vi "SetGain.vi"(10 "Gain":refnum<vi>, 11 ".NET Refnum in":refnum<k24>) -> (3 ".NET Refnum out":refnum<k24>)   [LabVIEW 2018]
uses:
  D:/SVN/PM/sdk/AppSamples/LabVIEWSamples/trunk/Release/2018/Dependencies/PVCamNET.dll
  Dependencies/PVCamNET.dll
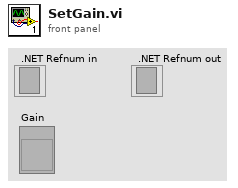
[diagram p1: front panel]
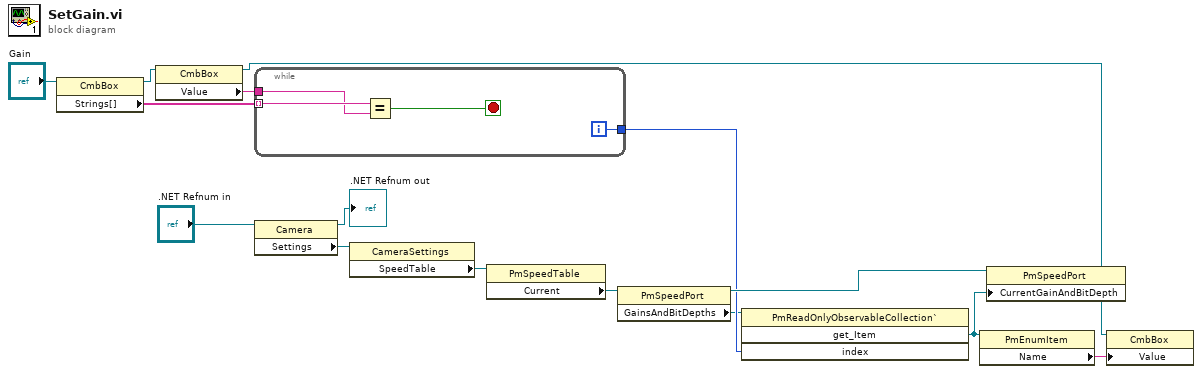
[diagram p0: block diagram]
diagram:
  n1 = property class="CmbBox"(reference="Gain") -> (reference out=w12:refnum<vi>, "Strings[]"=w3:string[])  [unwired: 1 in, 1 out]
  n2 = property class="CmbBox"(reference=w12) -> (reference out=w14:refnum<vi>, "Value"=w13:string)  [unwired: 1 in, 1 out]
  n3 = while {
    tunnel: w3 -> [w18] mode=indexing
    tunnel: [w17] -> w5
    tunnel: w13 -> [w16]
    i -> [w17]
    stop <- w19 stop-if-true
    n4 = Equal?(x=w18, y=w16) -> (x = y?=w19:bool)
  }
  n5 = property class="Camera"(reference=".NET Refnum in") -> (reference out=→".NET Refnum out":refnum<k24>, "Settings"=w1:refnum<k24>)  [unwired: 1 in, 1 out]
  n6 = property class="CameraSettings"(reference=w1) -> ("SpeedTable"=w10:refnum<k24>)  [unwired: 1 in, 2 out]
  n7 = property class="PmSpeedTable"(reference=w10) -> ("Current"=w7:refnum<k24>)  [unwired: 1 in, 2 out]
  n8 = property class="PmSpeedPort"(reference=w7) -> (reference out=w8:refnum<k24>, "GainsAndBitDepths"=w4:refnum<k24>)  [unwired: 1 in, 1 out]
  n9 = invoke class="PmReadOnlyObservableCollection`" method="get_Item"(reference=w4, "index"=w5) -> ("get_Item"=w9:refnum<k24>)  [unwired: 2 in, 3 out]
  n10 = property class="PmEnumItem"(reference=w9) -> ("Name"=w6:string)  [unwired: 1 in, 2 out]
  n11 = property class="PmSpeedPort"(reference=w8, "CurrentGainAndBitDepth"=w9) -> ()  [unwired: 1 in, 2 out]
  n12 = property class="CmbBox"(reference=w14, "Value"=w6) -> ()  [unwired: 1 in, 2 out]
